vi "Unsubscribe from Topic.vi"(8 "error in (no error)":errorcluster, 9 "Topic":string, 10 "Subscriber Enq":refnum<class "Message Enqueuer.lvclass">, 11 "Application Controller in":refnum<class "Application Controller.lvclass">) -> (0 "error out":errorcluster, 3 "Application Controller out":refnum<class "Application Controller.lvclass">)   [LabVIEW 2021, in "Application Controller.lvclass"]
uses:
  Application Controller.lvclass
  Application Controller.lvclass/Application Controller.ctl
  Publish-Subscribe/Interfaces/Publisher Messages/Unsubscribe from Topic Msg/Unsubscribe from Topic Msg.lvclass
  <vilib>/ActorFramework/Message Enqueuer/Message Enqueuer.lvclass
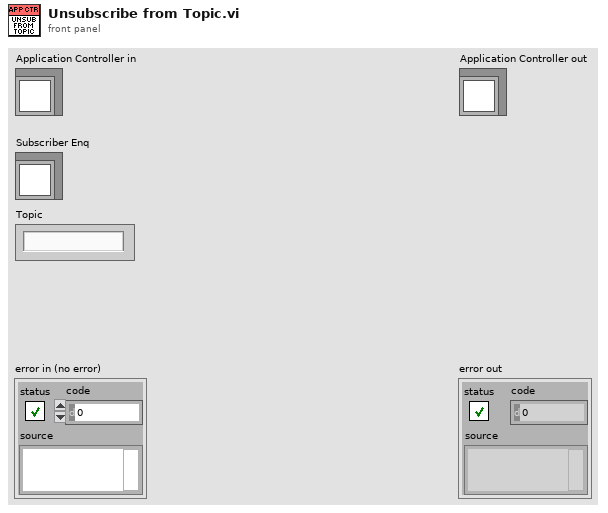
[diagram p1: front panel]
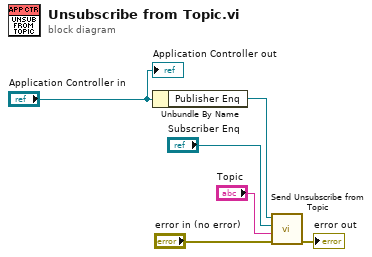
[diagram p0: block diagram]
diagram:
  n1 = Unbundle By Name("Application Controller in") -> ("Publisher Enq"=w5:refnum<class "Message Enqueuer.lvclass">)
  n2 = call "Send Unsubscribe from Topic.vi"("error in (no error)"="error in (no error)", "Topic"="Topic", "Subscriber Enq"="Subscriber Enq", "Message Enqueuer"=w5) -> ("error out"=→"error out":errorcluster)  [unwired: 6 in, 1 out]
  "Application Controller out" <- "Application Controller in"
